vi "PH_Tektronix_7000.Configure Trigger.vi"(0 "i ref in":refnum<vi>, 2 "Trigger Configuration":T1 {"Trigger Mode" items=["Normal", "Auto"]; "Coupling" items=["DC", "AC", "Hf Reject", "Lf Reject", "Noise Rej", "Atrigger"]; "Slope" items=["Rise", "Fall", "Either"]; "Source" items=["Channel1"=0, "Channel2"=1, "Channel3"=2, "Channel4"=3, "Aux"=12, "Line"=13]}, 5 "error IO":errorcluster) -> (14 "i ref out":refnum<vi>, 19 "error out":errorcluster)   [LabVIEW 2014, in "PH_Tektronix_7000.lvlib"]
doc: "If the connection is established, the trigger configuration is set and written to own attributes as well as the errors."
uses:
  PH_Tektronix_7000.lvlib
  PH_Tektronix_7000.Trigger Config.ctl
  non_GPL/instr.lib/Tektronix 7000 Series/Tektronix 7000 Series - Driver np.lvlib
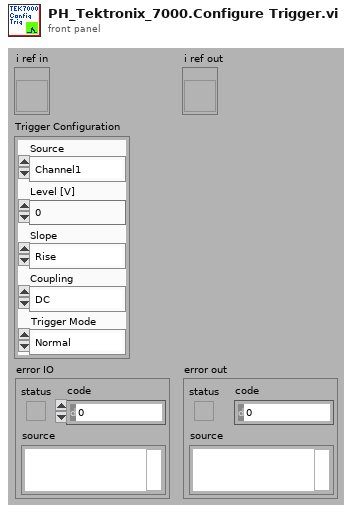
[diagram p1: front panel]
types:
  T1 = typedef "PH_Tektronix_7000.lvlib/PH_Tektronix_7000.Trigger Config.ctl" = cluster{"Source":u16, "Level [V]":dbl, "Slope":u16, "Coupling":u16, "Trigger Mode":u16}
  T2 = typedef "PH_Tektronix_7000.lvlib/PH_Tektronix_7000.i attribute.ctl" = cluster{"VISA Resource Name":refnum<visa-resource-name>, "IDN":cluster{"Instrument Driver":string, "Instrument Firmware":string, "Model":string, "Serial Number":string}, "Selftest":cluster{"Result":i32, "Message":string}, "Trigger Configuration":T1, "Acquisition Configuration":T3, "GUI Refs":T4, "State":T5, "Error Message":string, "Allow Prdc Loop?":bool, "Channel 1":T6, "Channel 2":T6, "Channel 3":T6, "Channel 4":T6, "Data CH 1":waveform(dbl), "Data CH 2":waveform(dbl), "Data CH 3":waveform(dbl), "Data CH 4":waveform(dbl), "Allow config?":bool, "Name Channel 1":string, "Name Channel 2":string, "Name Channel 3":string, "Name Channel 4":string, "Fetch Data before sending to PSDB?":bool, "Constructor passed?":bool, "Data taken at":timestamp, "Plot Colors":u32[], "Default VISA Resource":string}
  T3 = typedef "PH_Tektronix_7000.lvlib/PH_Tektronix_7000.Acquisition Config.ctl" = cluster{"Record Length":u32, "Timebase [s/div]":dbl, "Position [%]":dbl, "Acquisition Type":u16, "Average Waveforms":i32, "Envelope Waveforms":i32, "WfmDB Samples":i32, "Continuous?":bool, "Delay [s]":dbl, "Run?":bool}
  T4 = typedef "PH_Tektronix_7000.lvlib/PH_Tektronix_7000.GUI Refs.ctl" = cluster{"Graph":refnum<vi>, "State":refnum<vi>, "Delete":refnum<vi>, "VISA Resource":refnum<vi>, "Allow Configure":refnum<vi>, "Fetch Data":refnum<vi>, "Fetch before sending Data to PSDB":refnum<vi>, "Name Channel 1":refnum<vi>, "Name Channel 2":refnum<vi>, "Name Channel 3":refnum<vi>, "Name Channel 4":refnum<vi>, "Prdc Intervall [ms]":refnum<vi>, "Data taken":refnum<vi>, "Model":refnum<vi>, "Serial Number":refnum<vi>, "Firmware":refnum<vi>, "Driver":refnum<vi>, "Acquisition":refnum<vi>, "Trigger":refnum<vi>, "Cursor: D Time [s]":refnum<vi>, "Cursor: D Signal [V]":refnum<vi>, "Channel 1":refnum<vi>, "Channel 2":refnum<vi>, "Channel 3":refnum<vi>, "Channel 4":refnum<vi>}
  T5 = typedef "PH_StatusHandler.lvlib/PH_StatusHandler.Status.ctl" = i16
  T6 = typedef "PH_Tektronix_7000.lvlib/PH_Tektronix_7000.Channel Config.ctl" = cluster{"Enable Channel":bool, "Bandwidth":u16, "Input Impedance":u16, "Vertical Coupling":u16, "Probe Attenuation":dbl, "Range [V/div]":dbl, "Position [div]":dbl, "Bandwidth raw":string}
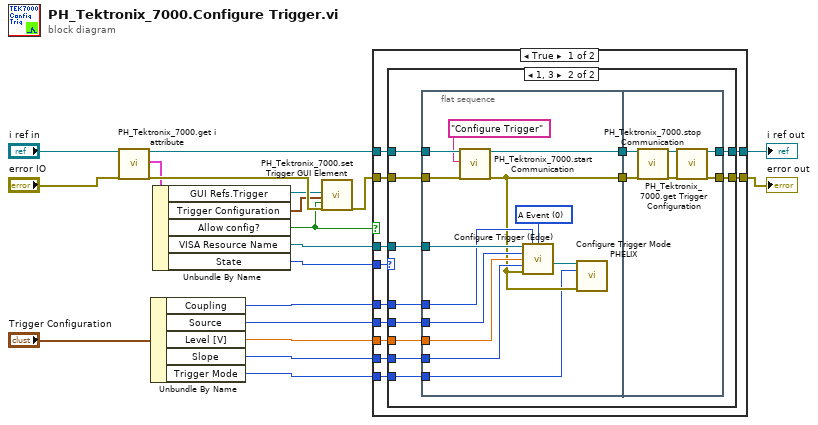
[diagram p0: block diagram]
diagram:
  n1 = call "PH_Tektronix_7000.get i attribute.vi"("i ref in"="i ref in", "error in (no error)"="error IO") -> ("i ref out"=w14:refnum<vi>, "i attribute"=w16:T2, "error out"=w18:errorcluster)  [unwired: 15 in]
  n2 = Unbundle By Name("Trigger Configuration") -> ("Coupling"=w11:u16, "Source"=w10:u16, "Level [V]"=w7:dbl, "Slope"=w6:u16, "Trigger Mode"=w1:u16)
  n3 = Unbundle By Name(w16) -> ("GUI Refs.Trigger"=w3:refnum<vi>, "Trigger Configuration"=w2:T1, "Allow config?"=w4:bool, "VISA Resource Name"=w17:refnum<visa-resource-name>, "State"=w9:T5)
  n4 = call "PH_Tektronix_7000.set Trigger GUI Element.vi"("Ref Trigger Config"=w3, "Trigger Config"=w2, "Enabled?"=w4, "error in"=w18) -> ("error out"=w5:errorcluster)  [unwired: 15 in]
  n5 = case shown="True" w4 {
    tunnel: [w30 w65] -> w19
    tunnel: w5 -> [w29 w64]
    tunnel: w17 -> [w28 _]
    tunnel: w14 -> [w27 w65]
    tunnel: [w26 w64] -> w12
    tunnel: w11 -> [w25 _]
    tunnel: w10 -> [w24 _]
    tunnel: w9 -> [w23 _]
    tunnel: w7 -> [w22 _]
    tunnel: w6 -> [w21 _]
    tunnel: w1 -> [w20 _]
    frame True {
      n6 = case shown="1, 3" w23 {
        tunnel: w27 -> [w32 w43]
        tunnel: w28 -> [_ w42]
        tunnel: [w31 w34] -> w26
        tunnel: w29 -> [w31 w44]
        tunnel: [w32 w35] -> w30
        tunnel: w25 -> [_ w41]
        tunnel: w24 -> [_ w40]
        tunnel: w22 -> [_ w39]
        tunnel: w21 -> [_ w38]
        tunnel: w20 -> [_ w33]
        frame Default {
        }
        frame 1, 3 {
          n7 = flat-sequence {
            tunnel: w44 -> [w57]
            tunnel: w43 -> [w56]
            tunnel: w42 -> [w54]
            tunnel: w41 -> [w48]
            tunnel: w40 -> [w53]
            tunnel: w39 -> [w52]
            tunnel: w38 -> [w51]
            tunnel: [w46] -> w37
            tunnel: [w49] -> w36
            tunnel: w33 -> [w45]
            tunnel: [w62] -> w35
            tunnel: [w61] -> w34
            tunnel: w37 -> [w59]
            tunnel: w36 -> [w63]
            frame #0 {
              w50 = u16 0 items=["A Event", "B Event"] ("Trigger Event (0:A Event)")
              n8 = call "PH_Tektronix_7000.start Communication.vi"("i ref in"=w56, "Action"="Configure Trigger", "error in"=w57) -> ("i ref out"=w49:refnum<vi>, "error out"=w46:errorcluster)  [unwired: 15 in]
              n9 = call "Configure Trigger (Edge).vi"("VISA resource name"=w54, "Coupling (0:DC)"=w48, "Trigger Event (0:A Event)"=w50, "Source (0:Channel1)"=w53, "Trigger Level (0.0V)"=w52, "Slope (0:Rise)"=w51, "error in (no error)"=w46) -> ("VISA resource name out"=w47:refnum<visa-resource-name>)  [unwired: 7 in, 1 out]
              n10 = call "Configure Trigger Mode PHELIX.vi"("VISA resource name"=w47, "Trigger Mode (0:Normal)"=w45, "error in (no error)"=w46) -> ()  [unwired: 11 in, 2 out]
            }
            frame #1 {
              n11 = call "PH_Tektronix_7000.stop Communication.vi"("i ref in"=w63, "error in"=w59) -> ("i ref out"=w60:refnum<vi>, "error out"=w58:errorcluster)  [unwired: 16 in]
              n12 = call "PH_Tektronix_7000.get Trigger Configuration.vi"("i ref in"=w60, "error IO"=w58) -> ("i ref out"=w62:refnum<vi>, "error out"=w61:errorcluster)  [unwired: 16 in]
            }
          }
        }
      }
    }
    frame False {
    }
  }
  "i ref out" <- w19
  "error out" <- w12
